vi "Replace Item Property.vi"(8 "error in (no error)":errorcluster, 9 "Replace Value":string, 10 "Replace Column":T1, 11 "Control in":refnum<class "Control.lvclass">) -> (0 "error out":errorcluster, 3 "Control out":refnum<class "Control.lvclass">)   [LabVIEW 2020, in "VI Properties Editor.lvlib" / "Control.lvclass"]
doc: "Replaces the value of the property identified by <B>Replace Column</B> with <B>Replace Value</B>."
uses:
  Control.lvclass
  CTLs/Replace Column.ctl
  VI Properties Editor.lvlib
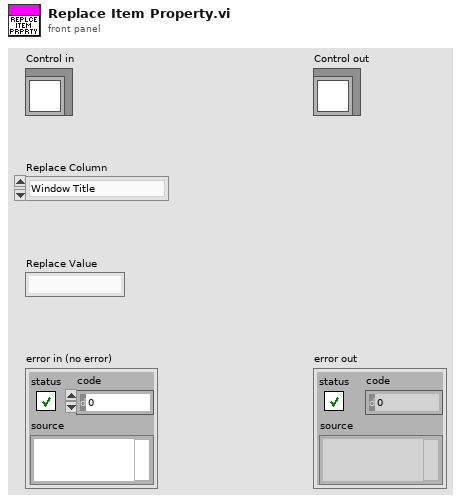
[diagram p1: front panel]
types:
  T1 = typedef "VI Properties Editor.lvlib/Replace Column.ctl" = enum16{"Window Title", "Description", "Help Path", "Help Tag", "Custom Title?", "Help URL", "Help Type", "Control Label", "Control Caption", "Control Description", "Control Tip Strip"}
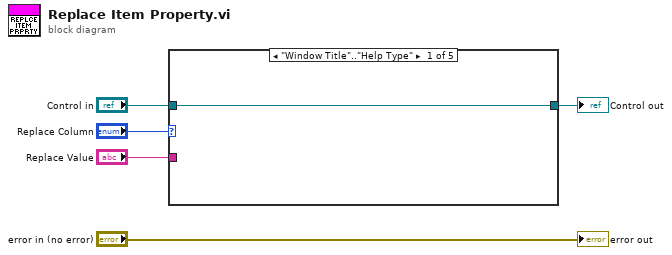
[diagram p0: block diagram]
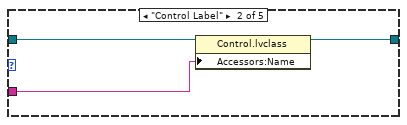
[diagram p2: hidden frame]
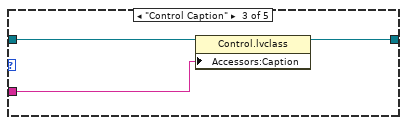
[diagram p3: hidden frame]
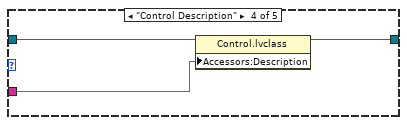
[diagram p4: hidden frame]
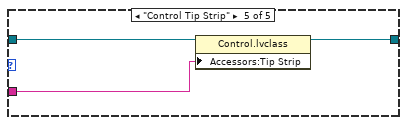
[diagram p5: hidden frame]
diagram:
  n1 = case shown="\"Window Title\"..\"Help Type\"" "Replace Column" {
    tunnel: "Control in" -> [w6 w9 w12 w15 w18]
    tunnel: [w6 w8 w11 w14 w17] -> w3
    tunnel: "Replace Value" -> [_ w7 w10 w13 w16]
    frame "Window Title".."Help Type" {
    }
    frame "Control Label" {
      n2 = property class="Control.lvclass"(reference=w9, "Accessors:Name"=w7) -> (reference out=w8:refnum<class "Control.lvclass">)  [unwired: 1 in, 1 out]
    }
    frame "Control Caption" {
      n3 = property class="Control.lvclass"(reference=w12, "Accessors:Caption"=w10) -> (reference out=w11:refnum<class "Control.lvclass">)  [unwired: 1 in, 1 out]
    }
    frame "Control Description" {
      n4 = property class="Control.lvclass"(reference=w15, "Accessors:Description"=w13) -> (reference out=w14:refnum<class "Control.lvclass">)  [unwired: 1 in, 1 out]
    }
    frame "Control Tip Strip" {
      n5 = property class="Control.lvclass"(reference=w18, "Accessors:Tip Strip"=w16) -> (reference out=w17:refnum<class "Control.lvclass">)  [unwired: 1 in, 1 out]
    }
  }
  "Control out" <- w3
  "error out" <- "error in (no error)"
